vi "Ignition Test.vi"(4 "Sequence Context":T1) -> (0 "error out":errorcluster, 1 "Test Data":T2 {"Numeric Measurement" format="%.2f"})   [LabVIEW 2012]
uses:
  <vilib>/addons/TestStand/_TSLegacy.llb/LabVIEW Test - Test Data.ctl
  <vilib>/addons/TestStand/_TSLegacy.llb/LabVIEW Test - Sequence Context.ctl
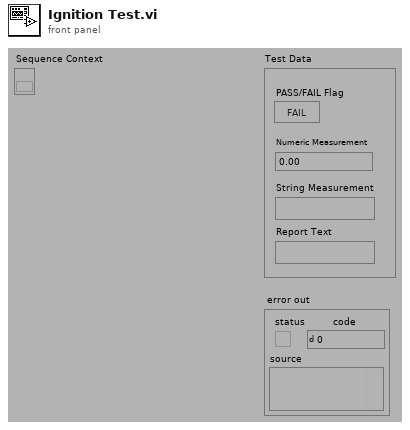
[diagram p1: front panel]
types:
  T1 = typedef "LabVIEW Test - Sequence Context.ctl" = refnum<k7>
  T2 = typedef "LabVIEW Test - Test Data.ctl" = cluster{"PASS/FAIL Flag":bool, "Numeric Measurement":dbl, "String Measurement":string, "Report Text":string}
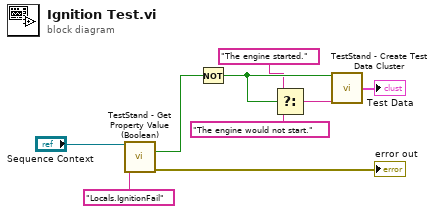
[diagram p0: block diagram]
diagram:
  n1 = call "TestStand - Get Property Value (Boolean).vi"("Sequence Context In"="Sequence Context", "Lookup String"="Locals.IgnitionFail") -> ("Value"=w5:bool, "error out"=→"error out":errorcluster)  [unwired: 1 in, 11 out]
  n2 = Not(x=w5) -> (.not. x?=w3:bool)
  n3 = Select(t="The engine started.", s=w3, f="The engine would not start.") -> (s? t:f=w4:string)
  n4 = call "TestStand - Create Test Data Cluster.vi"("Report Text"=w4, "PASS/FAIL Flag"=w3) -> ("Test Data"=→"Test Data":T2)  [unwired: 2 in]
